vi "PH_Cam_BaseClass.allocate or free img space.vi"(0 "i ref in":refnum<vi>, 2 "Allocate?":bool, 3 "Image Type":T1 {"Image Type" items=["Grayscale (U8)", "Grayscale (I16)", "Grayscale (SGL)", "Complex (CSG)", "RGB (U32)", "HSL (U32)", "RGB (U64)", "Grayscale (U16)"]}, 5 "error in (no error)":errorcluster) -> (14 "i ref out":refnum<vi>, 19 "error out":errorcluster)   [LabVIEW 2014, in "PH_Cam_BaseClass.lvlib"]
doc: "This VI is forseen to be used in constructor or destructor. If Allocate? = true is chosen, memory space for several images is allocated. If false is chosen, it is freed."
uses:
  PH_Cam_BaseClass.lvlib
  PH_Cam_BaseClass.Image Type.ctl
  CSCore/CSSystem/CSSystemLib/CSSystemLib.lvlib
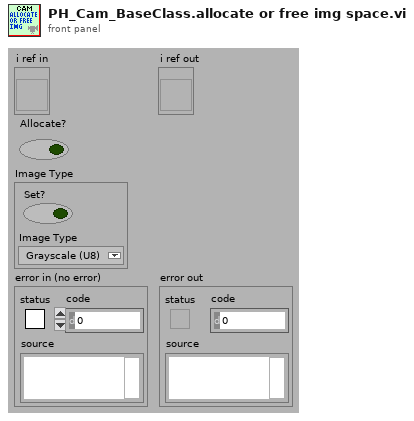
[diagram p1: front panel]
types:
  T1 = typedef "PH_Cam_BaseClass.lvlib/PH_Cam_BaseClass.Image Type.ctl" = cluster{"Set?":bool, "Image Type":T2}
  T2 = typedef "Image Type" = u32
  T3 = typedef "PH_Cam_BaseClass.lvlib/PH_Cam_BaseClass.i attribute.ctl" = cluster{"Gui Refs":T4, "Cam":cluster{"Source Notifier":refnum<notifier>, "Error":errorcluster, "Camera ID":string}, "Images":cluster{"Cam":T5, "Operation":T5, "PSDB":T5}, "Window Image":cluster{"Indicate Image":bool, "Window No.":i32, "Scale Facor":dbl, "Center Cross":bool, "Subtract Backgr":bool, "CoG":bool, "Color Palette":cluster{"Red":u8, "Green":u8, "Blue":u8}[], "Image On":bool}, "Default Prdc Int":i32, "Performance":cluster{"on":bool, "Timestamp Last Frame":i32}, "Histogram":cluster{"on":bool, "Mapping":bool}, "Save Image":cluster{"Save":bool, "File refnum":refnum<file>}, "Setting Service ID":i32, "Screen":cluster{"x-resolution":i16, "y-resolution":i16}, "On":bool, "Constructor finished":bool, "configured":bool}
  T4 = typedef "PH_Cam_BaseClass.lvlib/PH_Cam_BaseClass.GUI Refs.ctl" = cluster{"Frame Rate":refnum<vi>, "Get Frame Rate":refnum<vi>, "Show Image":refnum<vi>, "Get Histogram":refnum<vi>, "Mapping":refnum<vi>, "Histogram":refnum<vi>, "Center Cross":refnum<vi>, "Center of Gravity":refnum<vi>, "Scale Factor [%]":refnum<vi>, "Save Image":refnum<vi>, "Palette":refnum<vi>, "Subtract Background":refnum<vi>, "Cam Error":refnum<vi>, "On":refnum<vi>, "Cam List":refnum<vi>}
  T5 = typedef "IMAQ Image.ctl" = refnum<image>
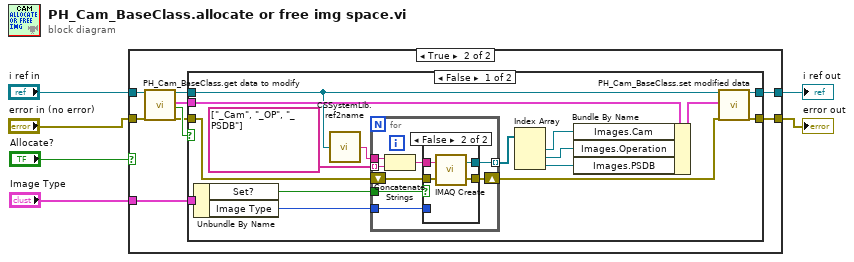
[diagram p0: block diagram]
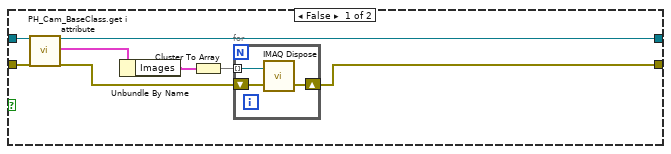
[diagram p2: hidden frame]
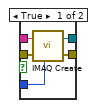
[diagram p3: hidden frame]
diagram:
  n1 = case shown="True" "Allocate?" {
    tunnel: [w9 w25] -> w6
    tunnel: [w11 w24] -> w5
    tunnel: "error in (no error)" -> [w14 w21]
    tunnel: "i ref in" -> [w13 w20]
    tunnel: "Image Type" -> [_ w18]
    frame False {
      n2 = call "PH_Cam_BaseClass.get i attribute.vi"("i ref in"=w13, "error in (no error)"=w14) -> ("i ref out"=w11:refnum<vi>, "i attribute"=w12:T3, "error out"=w10:errorcluster)  [unwired: 15 in]
      n3 = Unbundle By Name(w12) -> ("Images"=w8:cluster{"Cam":T5, "Operation":T5, "PSDB":T5})
      n4 = Cluster To Array(cluster=w8) -> (array=w7:T5[])
      n5 = for {
        shift-right: [w16] -> w9
        shift-left: w10 -> [w17]
        tunnel: w7 -> [w15] mode=indexing
        n6 = call "IMAQ Dispose"("Image"=w15, "error in (no error)"=w17) -> ("error out"=w16:errorcluster)  [unwired: 4 in]
      }
    }
    frame True {
      n7 = call "PH_Cam_BaseClass.get data to modify.vi"("i ref in"=w20, "error in (no error)"=w21) -> ("i ref out"=w23:refnum<vi>, "i attribute"=w19:T3, "timed out"=w26:bool, "error out"=w22:errorcluster)  [unwired: 14 in]
      n8 = case shown="False" w26 {
        tunnel: w22 -> [w33 w60]
        tunnel: w23 -> [w35 w61]
        tunnel: [w42 w61] -> w24
        tunnel: [w41 w60] -> w25
        tunnel: w19 -> [w36 _]
        tunnel: w18 -> [w29 _]
        frame False {
          n9 = Unbundle By Name(w29) -> ("Set?"=w28:bool, "Image Type"=w27:T2)
          n10 = call "CSSystemLib.ref2name.vi"("obj refnum"=w35) -> ("name"=w34:string)
          n11 = for {
            shift-right: [w50] -> w39
            shift-left: w33 -> [w49]
            tunnel: [w45] -> w38 mode=indexing
            tunnel: string[] ["_Cam", "_OP", "_PSDB"] -> [w47] mode=indexing
            tunnel: w34 -> [w48]
            tunnel: w28 -> [w44]
            tunnel: w27 -> [w43]
            n12 = Concatenate Strings(w48, w47) -> (w46:string)
            n13 = case shown="False" w44 {
              tunnel: [w55 w59] -> w50
              tunnel: w49 -> [w54 w58]
              tunnel: w46 -> [w53 w57]
              tunnel: [w52 w56] -> w45
              tunnel: w43 -> [w51 _]
              frame True {
                n14 = call "IMAQ Create"("Image Name"=w53, "Image Type"=w51, "error in (no error)"=w54) -> ("New Image"=w52:T5, "error out"=w55:errorcluster)  [unwired: 2 in]
              }
              frame False {
                n15 = call "IMAQ Create"("Image Name"=w57, "error in (no error)"=w58) -> ("New Image"=w56:T5, "error out"=w59:errorcluster)  [unwired: 3 in]
              }
            }
          }
          n16 = Index Array(array=w38) -> (element #1=w32:T5, element #2=w31:T5, element #3=w30:T5)  [unwired: 3 in]
          n17 = Bundle By Name(cluster=w36, "Images.Cam"=w32, "Images.Operation"=w31, "Images.PSDB"=w30) -> (w40:T3)
          n18 = call "PH_Cam_BaseClass.set modified data.vi"("i ref in"=w35, "i attribute"=w40, "error in (no error)"=w39) -> ("i ref out"=w42:refnum<vi>, "error out"=w41:errorcluster)  [unwired: 15 in]
        }
        frame True {
        }
      }
    }
  }
  "error out" <- w6
  "i ref out" <- w5
